vi "SubViTestTopLevel.vi"() -> ()   [LabVIEW 2014]
uses:
  <vilib>/rvi/Emulation/niFpgaGetClockAttributes.vi
  <vilib>/rvi/Emulation/niFpgaSctlEmulationGetInTimedLoop.vi
  <vilib>/rvi/Emulation/niFpgaEmulationReportErrorSimple.vi
  SubViTestGlobals.vi
  <vilib>/rvi/Emulation/niFpgaProcessEmulError.vi
  <vilib>/rvi/Emulation/niFpgaCriticalErrorInLSC.vi
panel:
  out "outerloops":i32
  in  "outerstop":bool
  out "0notPressed1Pressed":i16
  out "insideloop":i32
  in  "stop":bool
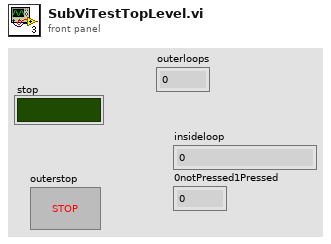
[diagram p1: front panel]
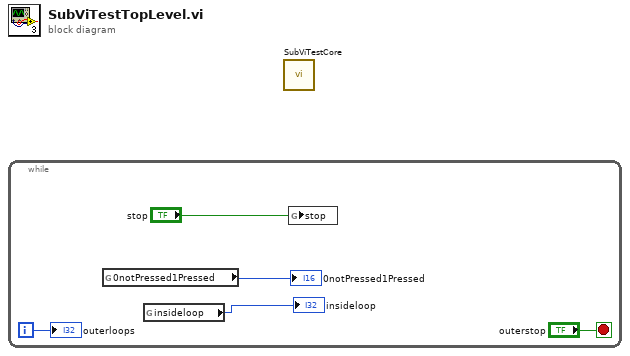
[diagram p0: block diagram]
diagram:
  n1 = while {
    i -> [w1]
    stop <- "outerstop" stop-if-true
    n2 = global read "SubViTestGlobals.vi" "0notPressed1Pressed"() -> (→"0notPressed1Pressed":i16)
    n3 = global read "SubViTestGlobals.vi" "insideloop"() -> (→"insideloop":i32)
    n4 = global write "SubViTestGlobals.vi" "stop"("stop") -> ()
    "outerloops" <- w1
  }
  n5 = call "SubViTestCore.vi"() -> ()  [unwired: 20 in]
